vi "Practica8_array.vi"() -> ()   [LabVIEW 2015]
uses:
  <vilib>/LabVIEW Interface for Arduino/LabVIEW Interface for Arduino.lvlib
panel:
  in  "Puerto Arduino":refnum<visa-resource-name>="COM6"
  in  "stop":bool
  out "Analog":dbl[](array[numeric])
  out "LED":bool[](array[boolean])
  in  "interruptores":bool[](array[boolean])
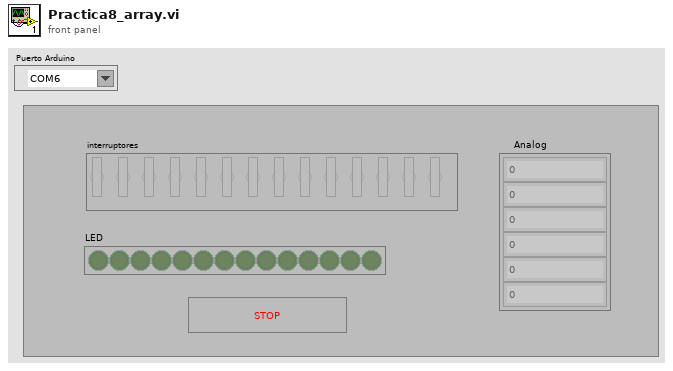
[diagram p1: front panel]
types:
  T1 = typedef "LabVIEW Interface for Arduino.lvlib/Arduino Resource.ctl" = cluster{"VISA resource":refnum<visa-resource-name>, "Board Type":T2, "Connection Type":enum8{"USB / Serial"}, "Bytes Per Packet (15)":u8}
  T2 = typedef "LabVIEW Interface for Arduino.lvlib/Board Type.ctl" = enum16{"Uno", "Dimuelanove w/Atmega 328", "Mega 2560"}
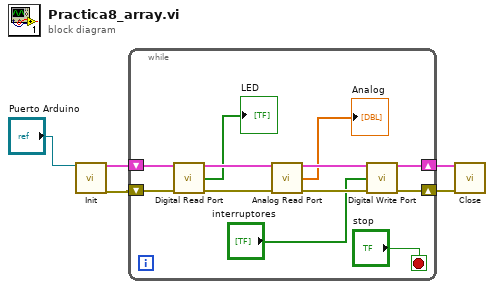
[diagram p0: block diagram]
diagram:
  n1 = call <vilib>:"Init.vi"("VISA resource"="Puerto Arduino") -> ("Arduino Resource"=w3:T1, "error out"=w2:errorcluster)  [unwired: 17 in]
  n2 = while {
    shift-right: [w12] -> w4
    shift-left: w3 -> [w11]
    shift-right: [w13] -> w5
    shift-left: w2 -> [w10]
    stop <- "stop" stop-if-true
    n3 = call <vilib>:"Digital Read Port.vi"("Arduino Resource"=w11, "error in"=w10) -> ("Arduino Resource"=w17:T1, "Digital Port"=→"LED":bool[], "error out"=w16:errorcluster)  [unwired: 11 in]
    n4 = call <vilib>:"Analog Read Port.vi"("Arduino Resource"=w17, "error in"=w16) -> ("Arduino Resource"=w14:T1, "Analog Port"=→"Analog":dbl[], "error out"=w15:errorcluster)  [unwired: 11 in]
    n5 = call <vilib>:"Digital Write Port.vi"("Arduino Resource"=w14, "Pin Values"="interruptores", "error in"=w15) -> ("Arduino Resource"=w12:T1, "error out"=w13:errorcluster)  [unwired: 11 in]
  }
  n6 = call <vilib>:"Close.vi"("Arduino Resource"=w4, "error in"=w5) -> ()  [unwired: 13 in, 1 out]
